vi "file operation status.vi"(8 "error in":errorcluster, 11 "File in":refnum<class "File.lvclass">) -> (0 "error out":errorcluster, 3 "String":string)   [LabVIEW 2023, in "File Classes.lvlib" / "File.lvclass"]
uses:
  File.lvclass
  File.lvclass/File.ctl
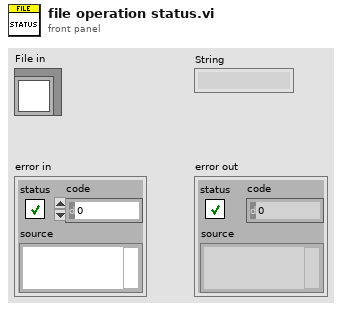
[diagram p1: front panel]
types:
  T1 = typedef "File Classes.lvlib/file operation enum.ctl" = enum16{"Copying", "Moving", "Deleting", "Skiped", "Renaming"}
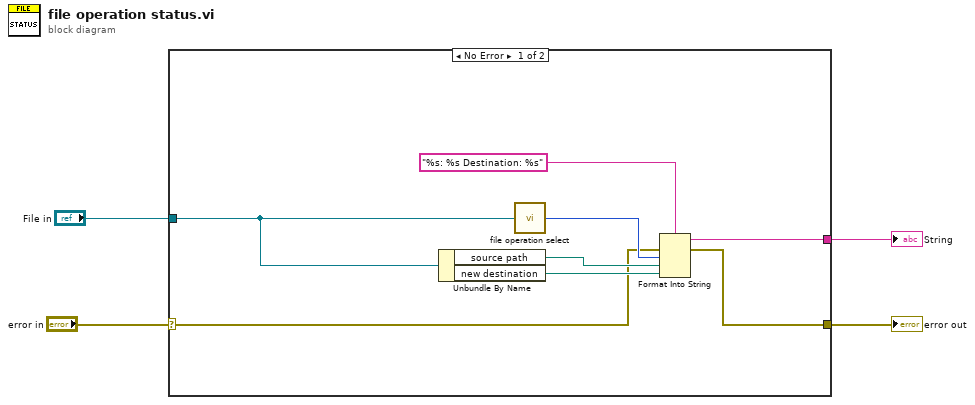
[diagram p0: block diagram]
diagram:
  n1 = case shown="No Error" "error in" {
    selector: "error in" -> [w8 w13]
    tunnel: [w7 w13] -> w3
    tunnel: "File in" -> [w6 _]
    tunnel: [w5 _] -> w1
    frame No Error {
      n2 = Unbundle By Name(w6) -> ("source path"=w12:path, "new destination"=w11:path)
      n3 = call "file operation select.vi"("File in"=w6) -> ("Operation"=w9:T1)
      n4 = Format Into String(format string="%s: %s Destination: %s", error in=w8, w9, w12, w11) -> (resulting string=w5:string, error out=w7:errorcluster)  [unwired: 1 in]
    }
    frame Error {
    }
  }
  "error out" <- w3
  "String" <- w1
